vi "Add PV Protocolls to FGV.vi"(8 "Error In":errorcluster, 10 "PV Protocol Section":string="PV_Protocols", 11 "CS++Factory":refnum<class "CS++Factory.lvclass">) -> (0 "Error Out":errorcluster)   [LabVIEW 2013, in "CS++ProcessVariables.lvlib"]
doc: "Read PV Protocols from configuration data to FGV."
uses:
  CS++ProcessVariables.lvlib
  CS++BaseClasses/Factory/CS++Factory.lvclass
  PVConnection/PVConnection.lvclass
  Libraries/Base/CS++Base.lvlib
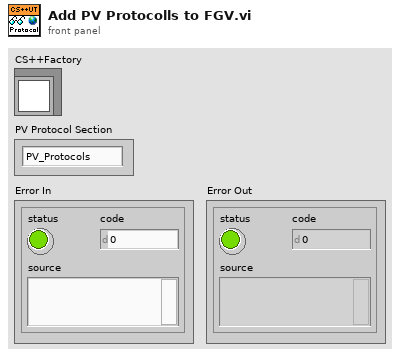
[diagram p1: front panel]
types:
  T1 = enum16{"add", "replace", "read", "remove", "reset", "get attibutes", ""}
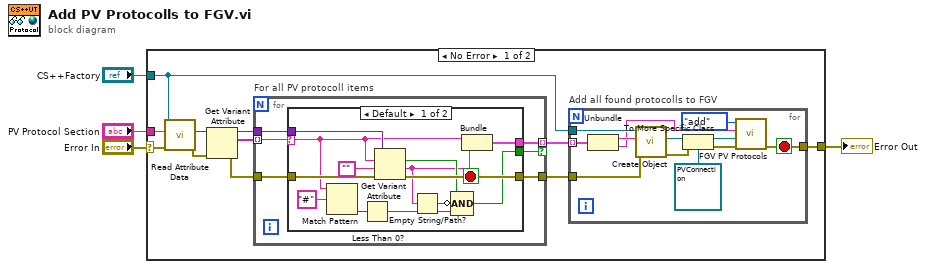
[diagram p0: block diagram]
diagram:
  n1 = case shown="No Error" "Error In" {
    selector: "Error In" -> [w5 w48]
    tunnel: "PV Protocol Section" -> [w8 _]
    tunnel: "CS++Factory" -> [w7 _]
    tunnel: [w6 w48] -> w2
    frame No Error {
      n2 = call-dynamic "Read Attribute Data.vi"("error in (no error)"=w5, "Object Name"=w8, "CS++Factory in"=w7) -> ("error out"=w15:errorcluster, "Attribute Data"=w14:variant)  [unwired: 6 in, 1 out]
      n3 = Get Variant Attribute(Variant=w14, error in=w15) -> (duplicate Variant=w12:variant, names=w13:string[], error out=w11:errorcluster)  [unwired: 2 in, 1 out]
      n4 = for "For all PV protocoll items" {
        tunnel: w13 -> [w28] mode=indexing
        tunnel: [w30] -> w9 mode=indexing if=w29
        tunnel: w12 -> [w33]
        tunnel: w11 -> [w32]
        tunnel: [w31] -> w10
        stop <- w31 stop-if-true
        n5 = case shown="Default" w28 {
          selector: w28 -> [w34 _]
          tunnel: w33 -> [w46 _]
          tunnel: w32 -> [w45 w47]
          tunnel: [w44 w47] -> w31
          tunnel: [w43 _] -> w30
          tunnel: [w42 _] -> w29
          frame Default {
            n6 = Match Pattern(string=w34, regular expression="#") -> (offset past match=w40:i32)  [unwired: 1 in, 3 out]
            n7 = Less Than 0?(x=w40) -> (x < 0?=w39:bool)
            n8 = Get Variant Attribute(Variant=w46, name=w34, default value (empty Variant)="", error in=w45) -> (found=w37:bool, value=w35:string, error out=w44:errorcluster)  [unwired: 1 out]
            n9 = Empty String/Path?(string/path=w35) -> (empty?=w36:bool)
            n10 = Compound Arithmetic op=AND(w37, invert w36, w39) -> (w42:bool)
            n11 = Bundle(w34, w35) -> (w43:cluster{string, string})  [unwired: 1 in]
          }
          frame "CS++ObjectName" {
          }
        }
      }
      n12 = for "Add all found protocolls to FGV" {
        tunnel: w10 -> [w22]
        tunnel: w9 -> [w27] mode=indexing
        tunnel: w7 -> [w25]
        tunnel: [w16] -> w6
        stop <- w16 stop-if-true
        n13 = Unbundle(w27) -> (w26:string, w18:string)
        n14 = call "Create Object.vi"("error in (no error)"=w22, "Object Name"=w26, "CS++Factory in"=w25) -> ("error out"=w23:errorcluster, "LabVIEW Object"=w24:refnum<class>)  [unwired: 5 in, 2 out]
        n15 = To More Specific Class(target class=refnum<class "PVConnection.lvclass"> refnum ("CS++ProcessVariables.lvlib:PVConnection.lvclass"), reference=w24, error in=w23) -> (specific class reference=w19:refnum<class "PVConnection.lvclass">, error out=w20:errorcluster)
        n16 = call "FGV PV Protocols.vi"("Error In"=w20, "PVConnection"=w19, "PV Protocoll"=w18, "Action (read)"=T1."add") -> ("Error Out"=w16:errorcluster)  [unwired: 3 in, 4 out]
      }
    }
    frame Error {
    }
  }
  "Error Out" <- w2
